vi "Keyence.Cmd.OperationCommands.Set.vi"(6 "Timeout [ms] (1000)":i32=1000, 8 "error in":errorcluster, 9 "Parameters":string, 10 "Cmd":T1, 11 "cID in":refnum<k5>) -> (0 "error out":errorcluster, 1 "OK?":bool, 2 "Response":string, 3 "cID out":refnum<k5>)   [LabVIEW 2016]
uses:
  Keyence.Cmd.OperationCommands.ctl
panel:
  out "response 2":string
  out "response 1":string
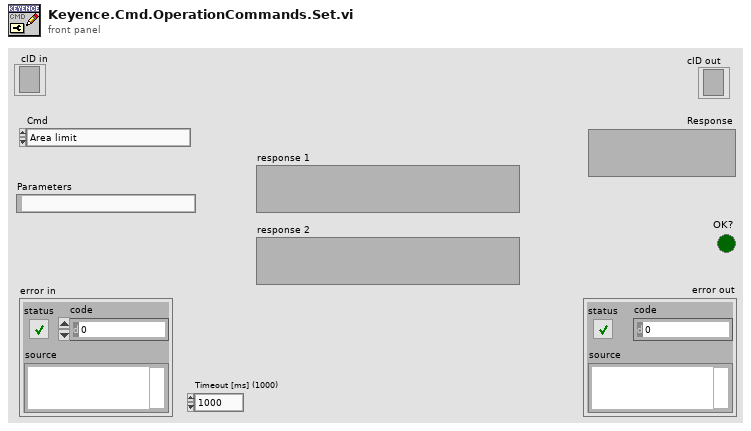
[diagram p1: front panel]
types:
  T1 = typedef "Keyence.Cmd.OperationCommands.ctl" = enum16{"Area limit"}
  T2 = enum16{"Standard", "Buffered", "CRLF", "Immediate"}
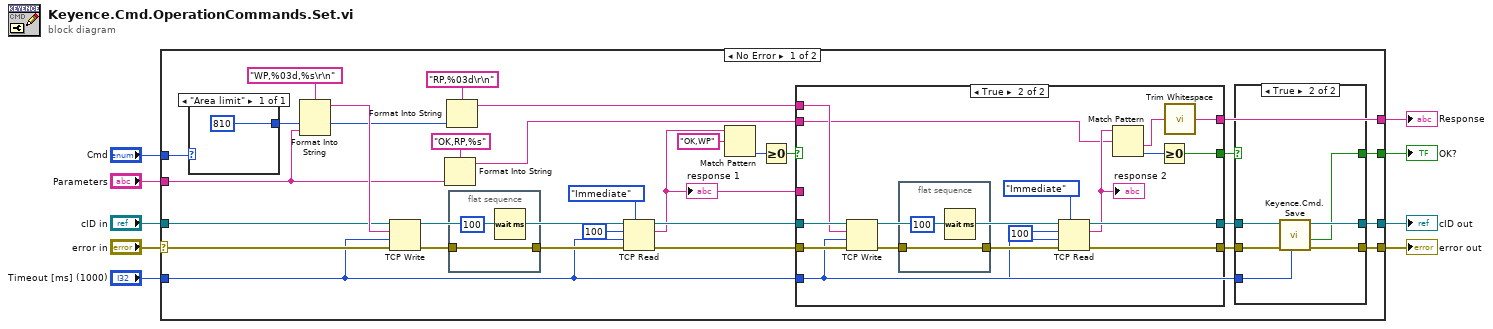
[diagram p0: block diagram]
diagram:
  n1 = case shown="No Error" "error in" {
    selector: "error in" -> [w28 w75]
    tunnel: "Timeout [ms] (1000)" -> [w12 _]
    tunnel: "Cmd" -> [w37 _]
    tunnel: "Parameters" -> [w17 _]
    tunnel: "cID in" -> [w29 w76]
    tunnel: [w16 w76] -> w4
    tunnel: [w15 w75] -> w1
    tunnel: [w19 _] -> w3
    tunnel: [w11 _] -> w2
    frame No Error {
      n2 = case shown="\"Area limit\"" w37 {
        tunnel: [810] -> w18
        frame "Area limit" {
        }
      }
      n3 = Format Into String(format string="WP,%03d,%s\r\n", w18, w17) -> (resulting string=w36:string)  [unwired: 2 in, 1 out]
      n4 = TCP Write(connection ID=w29, data in=w36, error in (no error)=w28, 9:w12) -> (connection ID out=w34:refnum<k5>, error out=w39:errorcluster)  [unwired: 1 out]
      n5 = Format Into String(format string="OK,RP,%s" ("regular expression"), w17) -> (resulting string=w20:string)  [unwired: 2 in, 1 out]
      n6 = Format Into String(format string="RP,%03d\r\n", w18) -> (resulting string=w26:string)  [unwired: 2 in, 1 out]
      n7 = flat-sequence {
        tunnel: w39 -> [w42]
        tunnel: [w42] -> w35
        frame #0 {
          n8 = Wait (ms)(milliseconds to wait=u32 100) -> ()  [unwired: 1 out]
        }
      }
      n9 = TCP Read(connection ID=w34, bytes to read=100, error in (no error)=w35, 7:T2."Immediate" ("mode (standard)"), 9:w12) -> (connection ID out=w32:refnum<k5>, data out=w30:string, error out=w33:errorcluster)
      "response 1" <- w30
      n10 = Match Pattern(string=w30, regular expression="OK,WP") -> (offset past match=w22:i32)  [unwired: 1 in, 3 out]
      n11 = Greater Or Equal To 0?(x=w22) -> (x >= 0?=w31:bool)
      n12 = case shown="True" w31 {
        selector: w31 -> [w43 _]
        tunnel: w33 -> [w45 w63]
        tunnel: w32 -> [w46 w62]
        tunnel: [w46 w52] -> w13
        tunnel: [w45 w53] -> w14
        tunnel: w12 -> [_ w55]
        tunnel: [w44 w47] -> w19
        tunnel: w30 -> [w44 _]
        tunnel: w26 -> [_ w61]
        tunnel: w20 -> [_ w49]
        tunnel: [w43 w50] -> w10
        frame False {
        }
        frame True {
          n13 = TCP Write(connection ID=w62, data in=w61, error in (no error)=w63, 9:w55) -> (connection ID out=w54:refnum<k5>, error out=w57:errorcluster)  [unwired: 1 out]
          n14 = flat-sequence {
            tunnel: w57 -> [w65]
            tunnel: [w65] -> w56
            frame #0 {
              n15 = Wait (ms)(milliseconds to wait=u32 100) -> ()  [unwired: 1 out]
            }
          }
          n16 = TCP Read(connection ID=w54, bytes to read=100, error in (no error)=w56, 7:T2."Immediate" ("mode (standard)"), 9:w55) -> (connection ID out=w52:refnum<k5>, data out=w51:string, error out=w53:errorcluster)
          "response 2" <- w51
          n17 = Match Pattern(string=w51, regular expression=w49) -> (after substring=w48:string, offset past match=w60:i32)  [unwired: 1 in, 2 out]
          n18 = Greater Or Equal To 0?(x=w60) -> (x >= 0?=w50:bool)
          n19 = call <vilib>:"Trim Whitespace.vi"("string"=w48) -> ("trimmed string"=w47:string)  [unwired: 1 in]
        }
      }
      n20 = case shown="True" w10 {
        selector: w10 -> [w66 _]
        tunnel: [w68 w74] -> w16
        tunnel: [w67 w73] -> w15
        tunnel: w14 -> [w67 w72]
        tunnel: w13 -> [w68 w71]
        tunnel: w12 -> [_ w70]
        tunnel: [w66 w69] -> w11
        frame False {
        }
        frame True {
          n21 = call "Keyence.Cmd.Save.vi"("Timeout [ms] (1000)"=w70, "error in"=w72, "cID in"=w71) -> ("error out"=w73:errorcluster, "OK?"=w69:bool, "cID out"=w74:refnum<k5>)  [unwired: 6 in]
        }
      }
    }
    frame Error {
    }
  }
  "cID out" <- w4
  "Response" <- w3
  "OK?" <- w2
  "error out" <- w1
